vi "Validate Arguments.vi"(8 "error in (no error)":errorcluster, 11 "UpdateAction in":refnum<class "UpdateAction.lvclass">) -> (0 "error out":errorcluster, 2 "Problems":string[](array[string]), 3 "UpdateAction out":refnum<class "UpdateAction.lvclass">)   [LabVIEW 2020, in "GPackTools.lvlib" / "UpdateAction.lvclass"]
uses:
  UpdateAction.lvclass
  UpdateAction.lvclass/UpdateAction.ctl
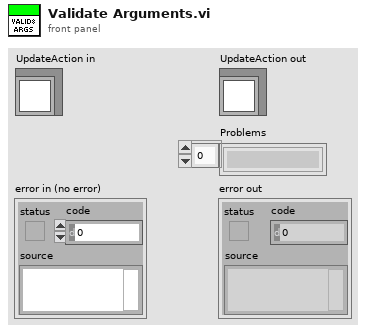
[diagram p1: front panel]
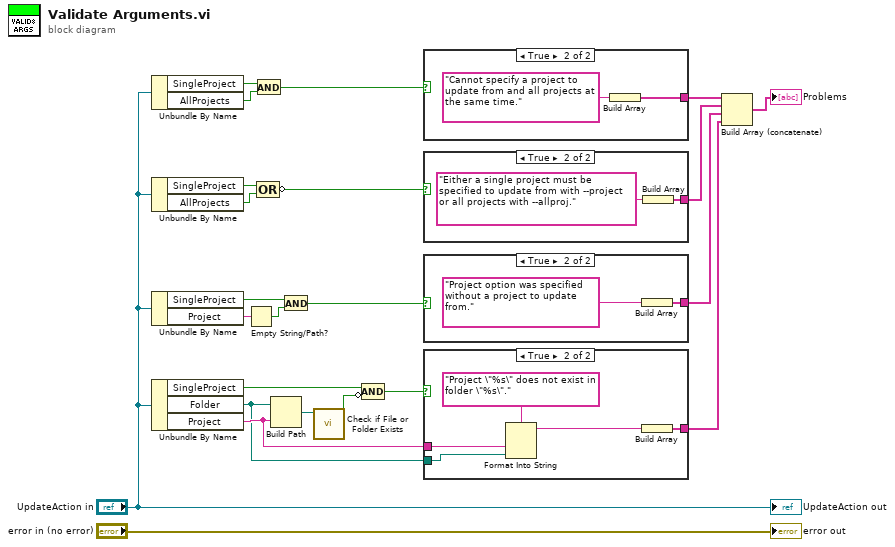
[diagram p0: block diagram]
diagram:
  n1 = Unbundle By Name("UpdateAction in") -> ("SingleProject"=w22:bool, "AllProjects"=w21:bool)
  n2 = Unbundle By Name("UpdateAction in") -> ("SingleProject"=w12:bool, "AllProjects"=w11:bool)
  n3 = Unbundle By Name("UpdateAction in") -> ("SingleProject"=w16:bool, "Project"=w17:string)
  n4 = Unbundle By Name("UpdateAction in") -> ("SingleProject"=w5:bool, "Folder"=w2:path, "Project"=w3:string)
  n5 = Empty String/Path?(string/path=w17) -> (empty?=w15:bool)
  n6 = And(x=w22, y=w21) -> (x .and. y?=w20:bool)
  n7 = Compound Arithmetic op=OR(w12, w11) -> (invert w10:bool)
  n8 = Build Path(base path=w2, name or relative path=w3) -> (appended path=w7:path)
  n9 = And(x=w16, y=w15) -> (x .and. y?=w14:bool)
  n10 = call <vilib>:"Check if File or Folder Exists.vi"("path"=w7) -> ("file or folder exists?"=w6:bool)  [unwired: 8 in, 2 out]
  n11 = Compound Arithmetic op=AND(w5, invert w6) -> (w4:bool)
  n12 = case shown="True" w20 {
    tunnel: [_ w24] -> w19
    frame False {
    }
    frame True {
      n13 = Build Array("Cannot specify a project to update from and all projects at the same time.") -> (w24:string[])
    }
  }
  n14 = case shown="True" w10 {
    tunnel: [_ w26] -> w9
    frame False {
    }
    frame True {
      n15 = Build Array("Either a single project must be specified to update from with --project or all projects with --allproj.") -> (w26:string[])
    }
  }
  n16 = case shown="True" w14 {
    tunnel: [_ w29] -> w13
    frame False {
    }
    frame True {
      n17 = Build Array("Project option was specified without a project to update from.") -> (w29:string[])
    }
  }
  n18 = case shown="True" w4 {
    tunnel: [_ w34] -> w1
    tunnel: w3 -> [_ w32]
    tunnel: w2 -> [_ w31]
    frame False {
    }
    frame True {
      n19 = Format Into String(format string="Project \"%s\" does not exist in folder \"%s\".", w32, w31) -> (resulting string=w30:string)  [unwired: 2 in, 1 out]
      n20 = Build Array(w30) -> (w34:string[])
    }
  }
  n21 = Build Array (concatenate)(w19, w9, w13, w1) -> (→"Problems":string[])
  "error out" <- "error in (no error)"
  "UpdateAction out" <- "UpdateAction in"
